vi "FGA Add Component to Node.vi"(1 "Node ID":u8, 2 "ComponentRec":T1={"Component Id"=1, "Instance Id"=0, "ServiceSeq"=[{"ServiceURI"="1", "MajorVerNum"=1, "MinorVerNum"=1}]}) -> (0 "Added?":bool)   [LabVIEW 2009]
uses:
  ComponentRec.ctl
  ServiceRec.ctl
  cRIO/Functional Global Variables/Actions for FG's.ctl
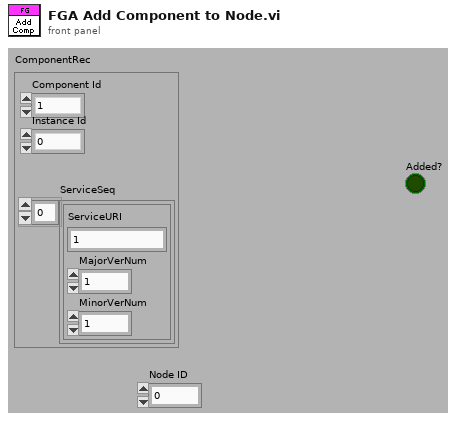
[diagram p1: front panel]
types:
  T1 = typedef "ComponentRec.ctl" = cluster{"Component Id":u8, "Instance Id":u8, "ServiceSeq":T2[]}
  T2 = typedef "ServiceRec.ctl" = cluster{"ServiceURI":string, "MajorVerNum":u8, "MinorVerNum":u8}
  T3 = typedef "NodeRec.ctl" = cluster{"Node Id":u8, "ComponentSeq":T1[]}
  T4 = typedef "Actions for FG's.ctl" = enum16{"Read", "Write"}
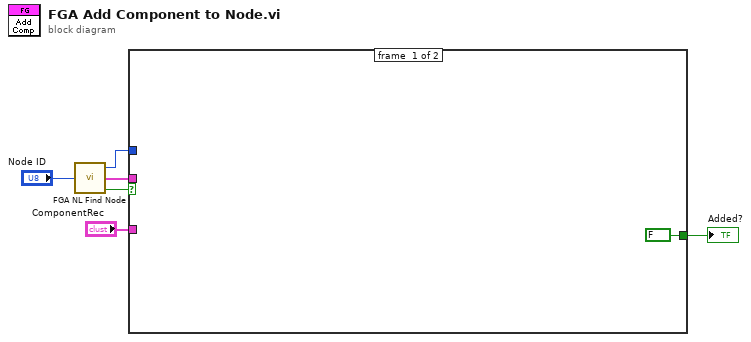
[diagram p0: block diagram]
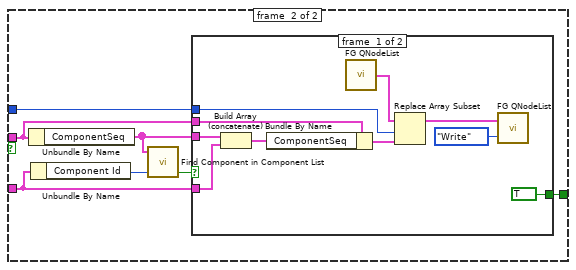
[diagram p2: hidden frame]
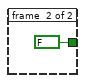
[diagram p3: hidden frame]
diagram:
  n1 = call "FGA NL Find Node.vi"("Node ID"="Node ID") -> ("Record Exists?"=w4:bool, "NodeRec"=w5:T3, "Node Index"=w2:i32)  [unwired: 2 in]
  n2 = case shown="True" w4 {
    tunnel: w5 -> [_ w9]
    tunnel: "ComponentRec" -> [_ w11]
    tunnel: w2 -> [_ w10]
    tunnel: [FALSE ("Boolean") w8] -> w1
    frame #0 {
    }
    frame #1 {
      n3 = Unbundle By Name(w9) -> ("ComponentSeq"=w12:T1[])
      n4 = Unbundle By Name(w11) -> ("Component Id"=w14:u8)
      n5 = call "Find Component in Component List.vi"("Component Id"=w14, "ComponentSeq"=w12) -> ("Record Exists?"=w13:bool)  [unwired: 1 in, 2 out]
      n6 = case shown="False" w13 {
        tunnel: w12 -> [w23 _]
        tunnel: w11 -> [w24 _]
        tunnel: w10 -> [w22 _]
        tunnel: w9 -> [w18 _]
        tunnel: [TRUE ("Boolean") FALSE ("Boolean")] -> w8
        frame #0 {
          n7 = Build Array (concatenate)(w23, w24) -> (w17:T1[])
          n8 = Bundle By Name(cluster=w18, "ComponentSeq"=w17) -> (w16:T3)
          n9 = call "FG QNodeList.vi"() -> ("NodeList out"=w21:T3[])  [unwired: 2 in]
          n10 = Replace Array Subset(array=w21, new element=w16, index=w22) -> (w19:T3[])
          n11 = call "FG QNodeList.vi"("FG Action (Read)"=Actions_for_FG's."Write", "NodeList in"=w19) -> ()  [unwired: 1 out]
        }
        frame #1 {
        }
      }
    }
  }
  "Added?" <- w1
